vi "Create Menus.vi"(8 "error in (no error)":errorcluster, 11 "Menu in":refnum<k9>) -> (0 "error out":errorcluster)   [LabVIEW 2017, in "DSF Configuration Utility.lvlib"]
uses:
  DSF Configuration Utility.lvlib
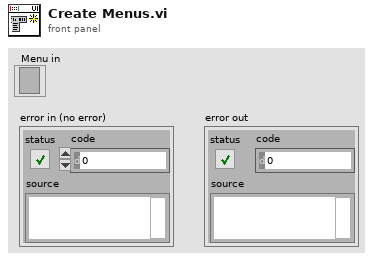
[diagram p1: front panel]
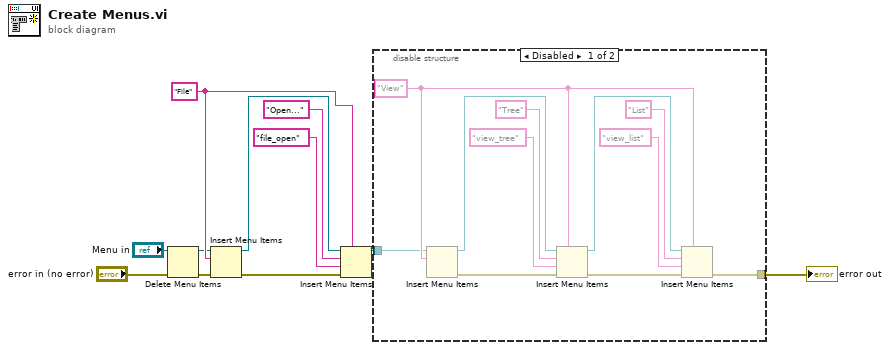
[diagram p0: block diagram]
diagram:
  w5 = "File" ("item names")
  n1 = Delete Menu Items(6:"error in (no error)", 9:"Menu in") -> (0:w10:errorcluster, 3:w2:refnum<k9>)  [unwired: 2 in]
  n2 = Insert Menu Items(6:w10, 8:w5, 9:w2) -> (0:w3:errorcluster, 3:w4:refnum<k9>)  [unwired: 3 in, 1 out]
  n3 = Insert Menu Items(5:w5, 6:w3, 7:"file_open" ("item tags"), 8:"Open..." ("item names"), 9:w4) -> (3:w8:refnum<k9>)  [unwired: 1 in, 2 out]
  n4 = disable-structure shown="Disabled" {
    disable-tunnel: [w22 _] -> w9
    disable-tunnel: w8 -> [w16 _]
    frame Disabled {
      w20 = "View" ("item names")
      n5 = Insert Menu Items(8:w20, 9:w16) -> (0:w15:errorcluster, 3:w14:refnum<k9>)  [unwired: 4 in, 1 out]
      n6 = Insert Menu Items(5:w20, 6:w15, 7:"view_tree" ("item tags"), 8:"Tree" ("item names"), 9:w14) -> (0:w21:errorcluster, 3:w19:refnum<k9>)  [unwired: 1 in, 1 out]
      n7 = Insert Menu Items(5:w20, 6:w21, 7:"view_list" ("item tags"), 8:"List" ("item names"), 9:w19) -> (0:w22:errorcluster)  [unwired: 1 in, 2 out]
    }
    frame Enabled {
    }
  }
  "error out" <- w9
